vi "Tosca-Update Adaptive Tracking.vi"(0 "Result":T3, 1 "Adapt":T4, 2 "Mode":T1, 7 "Abort? in":bool, 11 "error in (no error)":errorcluster, 12 "Analysis In":T8, 13 "Controls":T2) -> (4 "Finished":bool, 8 "Abort? out":bool, 14 "Analysis Out":T8, 15 "error out":errorcluster)   [LabVIEW 2020]
uses:
  Typedefs/Tosca-Analysis State.ctl
  Typedefs/Tosca-Adaptation State.ctl
  Typedefs/Tosca-Adaptation Track State.ctl
  Typedefs/Tosca-Adaptation History Element.ctl
  Classes/Parameters/Histogram Data.ctl
  Classes/Parameters/Connect.ctl
  Typedefs/Tosca-Adapt.ctl
  Typedefs/Tosca-Adaptive Track.ctl
  Typedefs/Tosca-Simple Variable.ctl
  Adaptation VIs/Tosca-Adapt Threshold Metric.ctl
  Typedefs/Tosca-Trial Result Enum.ctl
  Typedefs/Tosca-Control Refs.ctl
  FSM Graph VIs/LV Source/FSM Editor/FSM Editor.xctl
  Typedefs/Tosca-Schedule Mode.ctl
  Classes/Parameters/Parameters.lvclass
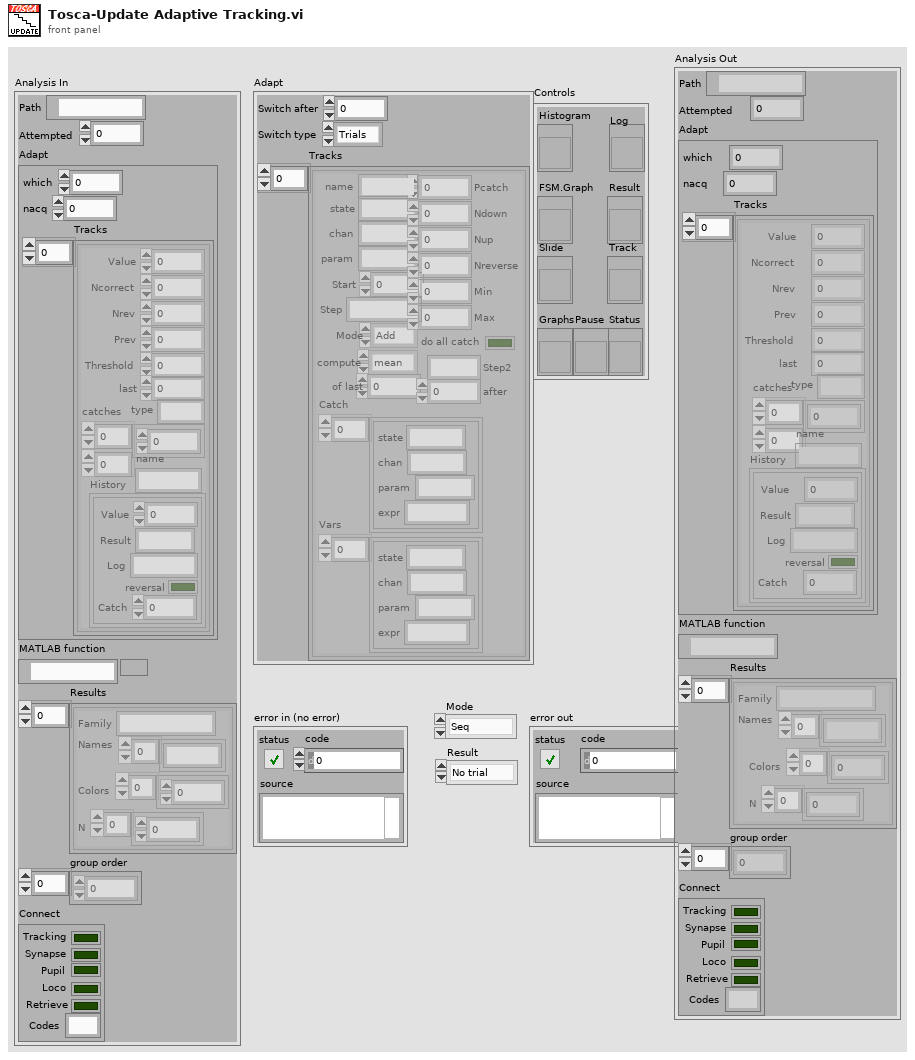
[diagram p1: front panel]
types:
  T1 = typedef "Tosca-Schedule Mode.ctl" = enum16{"Seq", "CS+/CS-", "Adapt"}
  T2 = typedef "Tosca-Control Refs.ctl" = cluster{"FSM.Graph":refnum<vi>, "Slide":refnum<vi>, "Result":refnum<vi>, "Histogram":refnum<vi>, "Graphs":refnum<vi>, "Track":refnum<vi>, "Log":refnum<vi>, "Status":refnum<vi>, "Pause":refnum<vi>}
  T3 = typedef "Tosca-Trial Result Enum.ctl" = enum16{"No trial", "Go", "No go", "Error", "Abort"}
  T4 = typedef "Tosca-Adapt.ctl" = cluster{"Switch after":i32, "Switch type":enum16{"Trials", "Reversals"}, "Tracks":T5[]}
  T5 = typedef "Tosca-Adaptive Track.ctl" = cluster{"state":string, "chan":string, "param":string, "Start":dbl, "Step":string, "Mode":enum16{"Add", "Multiply"}, "Pcatch":dbl, "Ndown":i32, "Nup":i32, "Nreverse":i32, "Min":dbl, "Max":dbl, "Catch":T6[], "do all catch":bool, "name":string, "Vars":T6[], "compute":T7, "of last":i32, "Step2":string, "after":i32}
  T6 = typedef "Tosca-Simple Variable.ctl" = cluster{"state":string, "chan":string, "param":string, "expr":string}
  T7 = typedef "Tosca-Adapt Threshold Metric.ctl" = enum16{"mean", "median"}
  T8 = typedef "Tosca-Analysis State.ctl" = cluster{"Path":path, "Attempted":i32, "Adapt":T9, "MATLAB function":path, "Results":T12[], "group order":i32[], "Connect":T13}
  T9 = typedef "Tosca-Adaptation State.ctl" = cluster{"which":i32, "nacq":i32, "Tracks":T10[]}
  T10 = typedef "Tosca-Adaptation Track State.ctl" = cluster{"Value":dbl, "Ncorrect":i32, "Nrev":i32, "Prev":dbl, "History":T11[], "Threshold":dbl, "last":i32, "type":string, "catches":dbl[][], "name":string}
  T11 = typedef "Tosca-Adaptation History Element.ctl" = cluster{"Value":dbl, "Result":string, "Log":string, "reversal":bool, "Catch":dbl}
  T12 = typedef "Parameters.lvclass/Histogram Data.ctl" = cluster{"Family":string, "Names":string[], "Colors":u32[], "N":i32[]}
  T13 = typedef "Parameters.lvclass/Connect.ctl" = cluster{"Tracking":bool, "Synapse":bool, "Pupil":bool, "Loco":bool, "Retrieve":bool, "Codes":string}
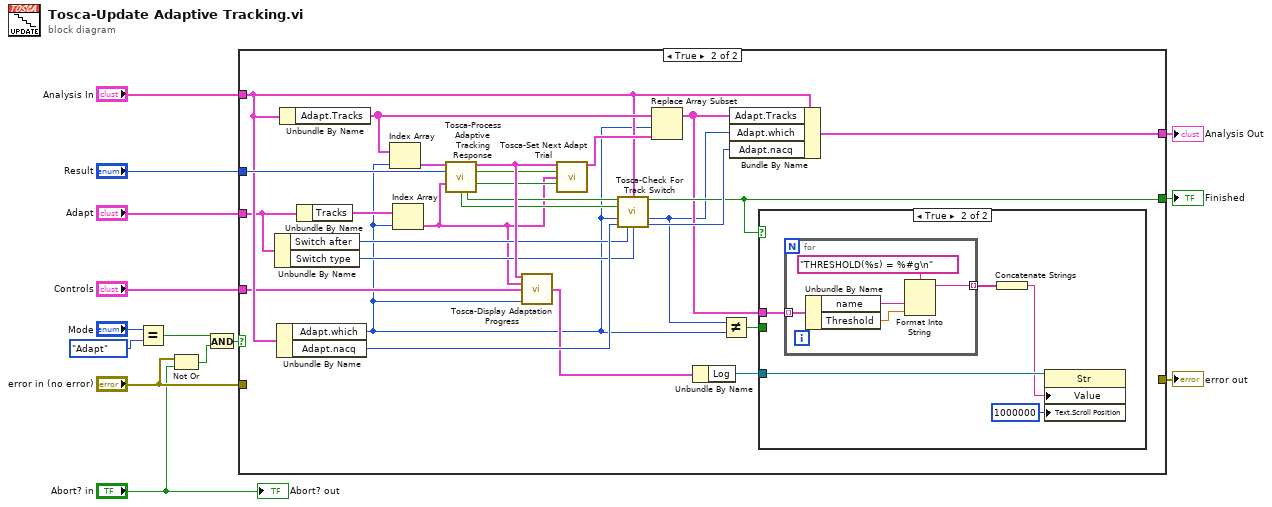
[diagram p0: block diagram]
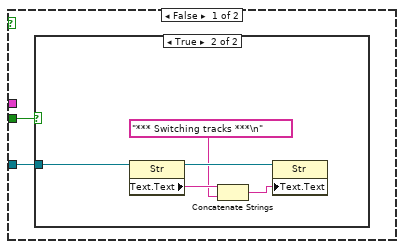
[diagram p3: hidden frame]
diagram:
  n1 = Equal?(x="Mode", y=Tosca-Schedule_Mode."Adapt") -> (x = y?=w2:bool)
  n2 = Not Or(1:"Abort? in", 2:"error in (no error)") -> (0:w8:bool)
  n3 = And(x=w2, y=w8) -> (x .and. y?=w7:bool)
  n4 = case shown="True" w7 {
    tunnel: "Adapt" -> [_ w30]
    tunnel: "Analysis In" -> [w16 w35]
    tunnel: [w16 w38] -> w13
    tunnel: [w15 _] -> w14
    tunnel: "error in (no error)" -> [w15 _]
    tunnel: "Result" -> [_ w42]
    tunnel: "Controls" -> [_ w25]
    tunnel: [_ w27] -> w5
    frame False {
    }
    frame True {
      n5 = Unbundle By Name(w30) -> ("Switch after"=w29:i32, "Switch type"=w28:enum16{"Trials", "Reversals"})
      n6 = Unbundle By Name(w35) -> ("Adapt.which"=w21:i32, "Adapt.nacq"=w31:i32)
      n7 = Unbundle By Name(w35) -> ("Adapt.Tracks"=w39:T10[])
      n8 = Unbundle By Name(w30) -> ("Tracks"=w41:T5[])
      n9 = Index Array(array=w39, index=w21) -> (element=w40:T10)
      n10 = Index Array(array=w41, index=w21) -> (element=w17:T5)
      n11 = call "Tosca-Process Adaptive Tracking Response.vi"("Track in"=w40, "Result"=w42, "Track"=w17) -> ("Track out"=w37:T10, "change"=w19:bool, "catch is tracked"=w18:bool, "reversal"=w33:bool, "Finished"=w34:bool)  [unwired: 8 in]
      n12 = call "Tosca-Display Adaptation Progress.vi"("Track"=w37, "Track def"=w17, "Controls"=w25, "which"=w21) -> ("Controls thru"=w23:T2)  [unwired: 11 in]
      n13 = call "Tosca-Set Next Adapt Trial.vi"("Track in"=w37, "change"=w19, "Track"=w17, "catch is tracked"=w18) -> ("Track out"=w36:T10)  [unwired: 11 in]
      n14 = call "Tosca-Check For Track Switch.vi"("Finished in"=w34, "Analysis In"=w35, "reversal"=w33, "which in"=w21, "nacq"=w31, "Switch after"=w29, "Switch type"=w28) -> ("Finished out"=w27:bool, "which out"=w22:i32, "nacq out"=w32:i32)  [unwired: 6 in]
      n15 = Replace Array Subset(array=w39, new element=w36, index=w21) -> (w26:T10[])
      n16 = Unbundle By Name(w23) -> ("Log"=w24:refnum<vi>)
      n17 = Not Equal?(x=w22, y=w21) -> (x != y?=w20:bool)
      n18 = Bundle By Name(cluster=w35, "Adapt.Tracks"=w26, "Adapt.which"=w22, "Adapt.nacq"=w32) -> (w38:T8)
      n19 = case shown="True" w27 {
        tunnel: w26 -> [_ w54]
        tunnel: w24 -> [w44 w52]
        tunnel: w20 -> [w43 _]
        frame False {
          n20 = case shown="True" w43 {
            tunnel: w44 -> [_ w49]
            frame False {
            }
            frame True {
              n21 = property class="Str"(reference=w49) -> (reference out=w47:refnum<vi>, "Text.Text"=w48:string)  [unwired: 1 in, 1 out]
              n22 = Concatenate Strings(w48, "*** Switching tracks ***\n") -> (w46:string)
              n23 = property class="Str"(reference=w47, "Text.Text"=w46) -> ()  [unwired: 1 in, 2 out]
            }
          }
        }
        frame True {
          n24 = for {
            tunnel: w54 -> [w59] mode=indexing
            tunnel: [w56] -> w51 mode=indexing
            n25 = Unbundle By Name(w59) -> ("name"=w55:string, "Threshold"=w57:dbl)
            n26 = Format Into String(format string="THRESHOLD(%s) = %#g\n", w55, w57) -> (resulting string=w56:string)  [unwired: 2 in, 1 out]
          }
          n27 = Concatenate Strings(w51) -> (w50:string)
          n28 = property class="Str"(reference=w52, "Value"=w50, "Text.Scroll Position"=u32 1000000) -> ()  [unwired: 1 in, 2 out]
        }
      }
    }
  }
  "Finished" <- w5
  "error out" <- w14
  "Analysis Out" <- w13
  "Abort? out" <- "Abort? in"
